vi "Measure the Function on 2nd Display.vi"(7 "Manual Range":dbl format="%#.9e", 8 "error in":errorcluster, 9 "Enable Auto Range":bool=TRUE, 10 "Function":u8(ring) items=["DC Voltage", "AC Voltage", "DC Current", "AC Current", "2-Wire Resistance", "Frequency", "Period"], 11 "VISA resource name":refnum<visa-resource-name>) -> (0 "error out":errorcluster, 2 "Return the Value":string, 3 "VISA resource name out":refnum<visa-resource-name>)   [LabVIEW 2011, in "DMM4.lvlib"]
uses:
  <instrlib>/DMM4/DMM4.lvlib
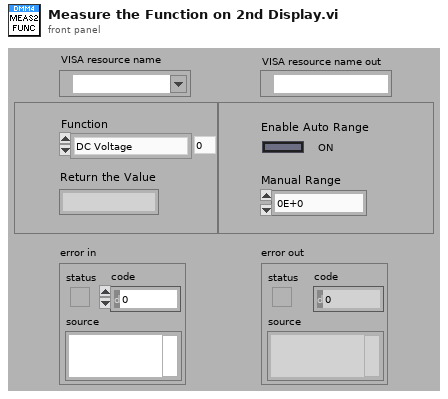
[diagram p1: front panel]
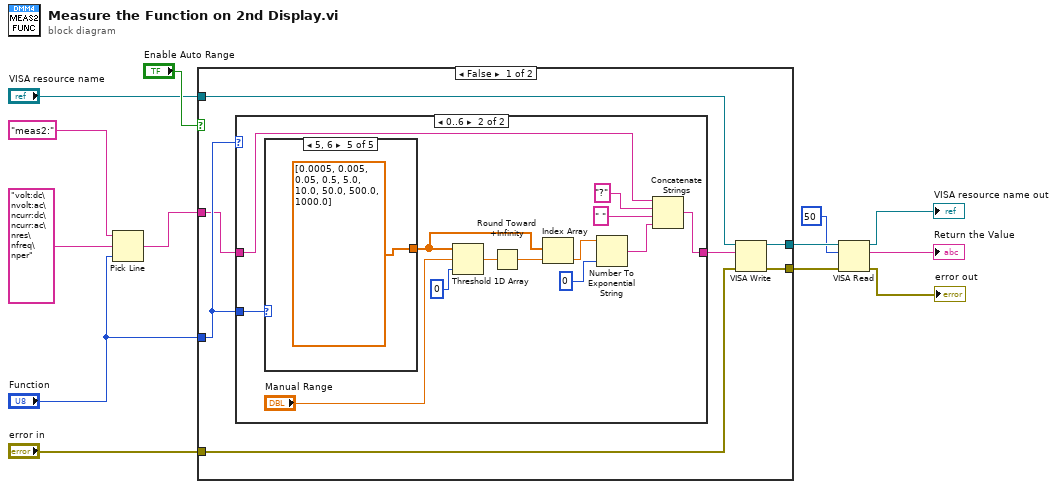
[diagram p0: block diagram]
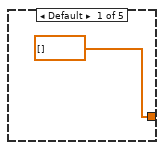
[diagram p3: hidden frame]
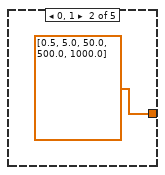
[diagram p4: hidden frame]
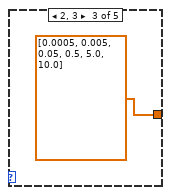
[diagram p5: hidden frame]
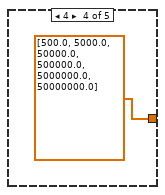
[diagram p6: hidden frame]
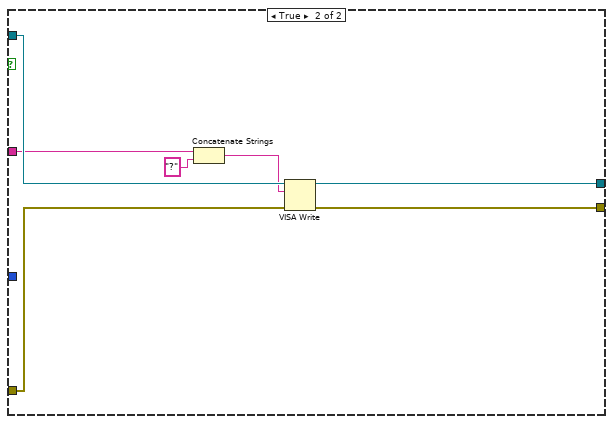
[diagram p7: hidden frame]
diagram:
  n1 = Pick Line(string ("")="meas2:", multi-line string="volt:dc\nvolt:ac\ncurr:dc\ncurr:ac\nres\nfreq\nper", line index="Function") -> (output string=w9:string)
  n2 = case shown="False" "Enable Auto Range" {
    tunnel: "Function" -> [w20 _]
    tunnel: w9 -> [w19 w41]
    tunnel: "VISA resource name" -> [w17 w46]
    tunnel: "error in" -> [w16 w45]
    tunnel: [w15 w44] -> w6
    tunnel: [w14 w43] -> w5
    frame False {
      n3 = case shown="0..6" w20 {
        tunnel: w20 -> [_ w25]
        tunnel: w19 -> [w21 w27]
        tunnel: [w21 w26] -> w18
        frame Default {
        }
        frame 0..6 {
          n4 = case shown="5, 6" w25 {
            tunnel: [dbl[] [] dbl[] [0.5, 5.0, 50.0, 500.0, 1000.0] dbl[] [0.0005, 0.005, 0.05, 0.5, 5.0, 10.0] dbl[] [500.0, 5000.0, 50000.0, 500000.0, 5000000.0, 50000000.0] dbl[] [0.0005, 0.005, 0.05, 0.5, 5.0, 10.0, 50.0, 500.0, 1000.0]] -> w30
            frame Default {
            }
            frame 0, 1 {
            }
            frame 2, 3 {
            }
            frame 4 {
            }
            frame 5, 6 {
            }
          }
          n5 = Threshold 1D Array(1:0 ("start index (0)"), 2:"Manual Range", 3:w30) -> (0:w32:dbl)
          n6 = Round Toward +Infinity(x=w32) -> (ceil(x): smallest int >= x=w31:dbl)
          n7 = Index Array(array=w30, index=w31) -> (element=w29:dbl)
          n8 = Number To Exponential String(number=w29, precision (6)=i16 0) -> (E-format string=w22:string)  [unwired: 2 in]
          n9 = Concatenate Strings(w27, "?" ("string"), " " ("string"), w22) -> (w26:string)
        }
      }
      n10 = VISA Write(VISA resource name=w17, write buffer=w18, error in (no error)=w16) -> (VISA resource name out=w15:refnum<visa-resource-name>, error out=w14:errorcluster)  [unwired: 1 out]
    }
    frame True {
      n11 = Concatenate Strings(w41, "?" ("string")) -> (w40:string)
      n12 = VISA Write(VISA resource name=w46, write buffer=w40, error in (no error)=w45) -> (VISA resource name out=w44:refnum<visa-resource-name>, error out=w43:errorcluster)  [unwired: 1 out]
    }
  }
  n13 = VISA Read(VISA resource name=w6, byte count=u32 50, error in (no error)=w5) -> (VISA resource name out=→"VISA resource name out":refnum<visa-resource-name>, read buffer=→"Return the Value":string, error out=→"error out":errorcluster)  [unwired: 1 out]
